vi "ProdaNG.Tree.Clear.vi"(7 "TestStepsTree":refnum<vi>, 8 "error in (no error)":errorcluster) -> (0 "error out":errorcluster)   [LabVIEW 2016]
uses:
  ProdaNG.Tree.Fglb.Action.ctl
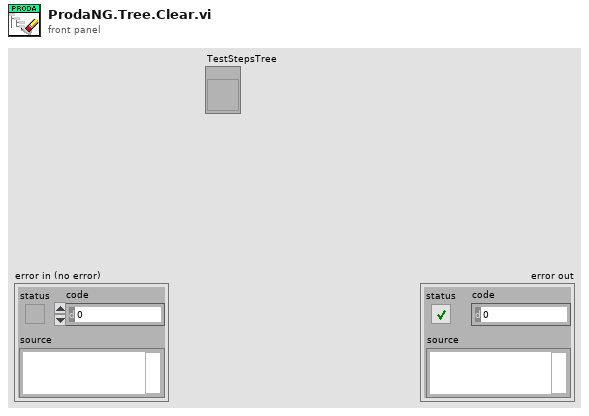
[diagram p1: front panel]
types:
  T1 = typedef "ProdaNG.Tree.Fglb.Action.ctl" = enum16{"init", "add", "get by row", "get by tag", "get by idx"}
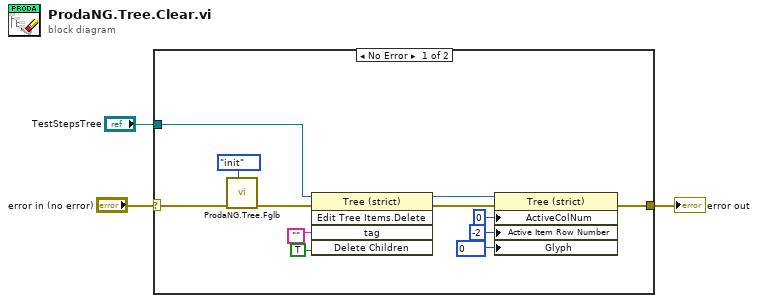
[diagram p0: block diagram]
diagram:
  n1 = case shown="No Error" "error in (no error)" {
    selector: "error in (no error)" -> [w8 w16]
    tunnel: "TestStepsTree" -> [w15 _]
    tunnel: [w10 w16] -> w3
    frame No Error {
      n2 = call "ProdaNG.Tree.Fglb.vi"("Action (add)"=ProdaNG.Tree.Fglb.Action."init", "error in"=w8) -> ("error out"=w7:errorcluster)  [unwired: 7 in, 2 out]
      n3 = invoke on="Invoke Node" class="Tree (strict)" method="Edit Tree Items.Delete"(reference=w15, error in=w7, "tag"="", "Delete Children"=TRUE ("Delete Children?")) -> (reference out=w11:refnum<vi>, error out=w12:errorcluster)  [unwired: 1 in, 3 out]
      n4 = property class="Tree (strict)"(reference=w11, error in=w12, "ActiveColNum"=0 ("Active Cell:Active Column Number"), "Active Item Row Number"=-2 ("Active Item:Row Number"), "Glyph"=0) -> (error out=w10:errorcluster)  [unwired: 1 out]
    }
    frame Error {
    }
  }
  "error out" <- w3
